vi "Create GUI Element.vi"(8 "error in (no error)":errorcluster, 10 "Highlight index":i32=-1, 11 "Sequence of SBlocks in":refnum<class "Sequence of SBlocks.lvclass">) -> (0 "error out":errorcluster, 2 "Sequence of SBlocks - GUI":T1, 3 "Sequence of SBlocks out":refnum<class "Sequence of SBlocks.lvclass">)   [LabVIEW 2020, in "TALOS.lvlib" / "Run Utilities.lvlib" / "Sequence of SBlocks.lvclass"]
uses:
  Sequence of SBlocks.lvclass
  Sequence of SBlcoks - GUI.ctl
  Schedule Block/Schedule Block - simplified GUI.ctl
  Sequence of SBlocks.lvclass/Sequence of SBlocks.ctl
  Schedule Block/Schedule Block.lvclass
panel:
  # "Estimated time of execution"
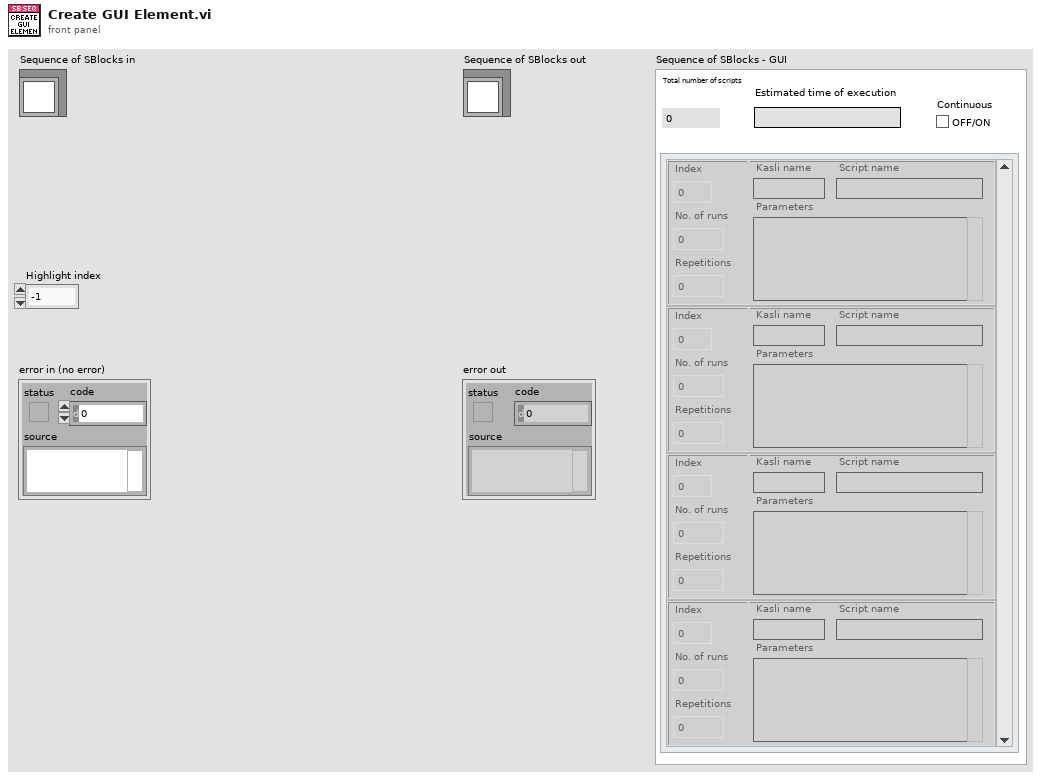
[diagram p1: front panel]
types:
  T1 = typedef "TALOS.lvlib/Run Utilities.lvlib/Sequence of SBlocks.lvclass/Sequence of SBlcoks - GUI.ctl" = cluster{"Total number of scripts":i32, "Time":string, "Sequence of SBlocks":T2[], "Continuous":bool}
  T2 = typedef "TALOS.lvlib/Run Utilities.lvlib/Schedule Block.lvclass/Schedule Block - simplified GUI.ctl" = cluster{"Bcg Color":u32, "Index":i32, "No. of runs":i32, "Script name":string, "Kasli name":string, "Parameters":string, "Repetitions":i32}
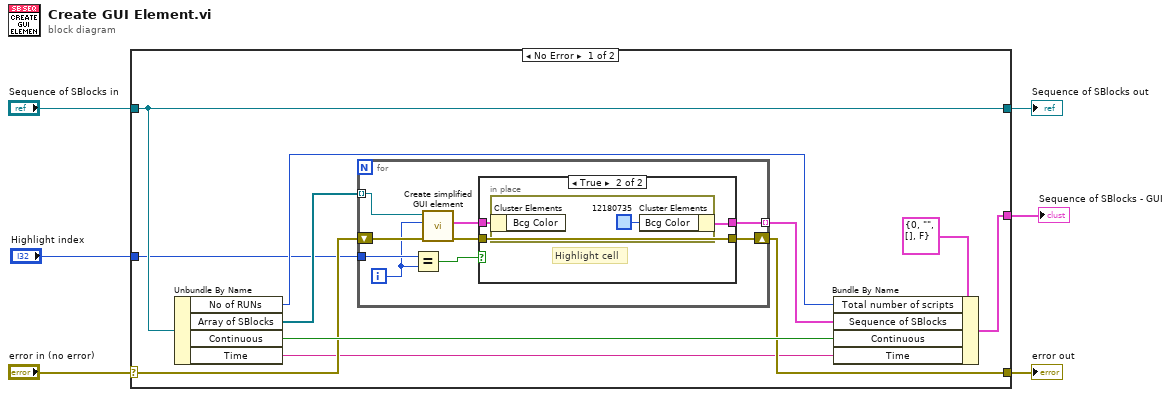
[diagram p0: block diagram]
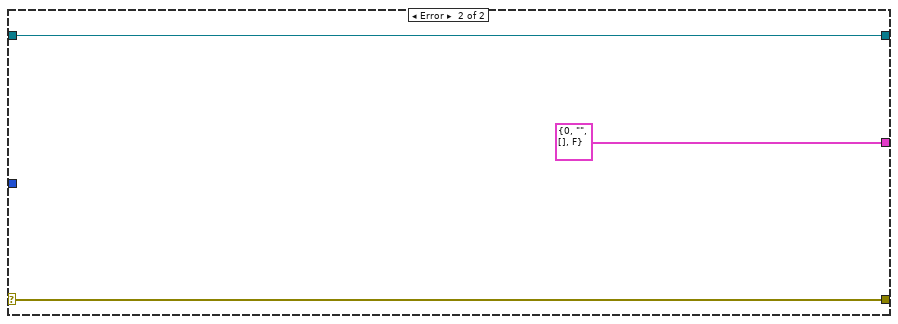
[diagram p3: hidden frame]
diagram:
  n1 = case shown="No Error" "error in (no error)" {
    selector: "error in (no error)" -> [w11 w35]
    tunnel: [w10 w35] -> w5
    tunnel: [w17 w34] -> w3
    tunnel: "Sequence of SBlocks in" -> [w17 w34]
    tunnel: [w12 T1 {"Total number of scripts"=0, "Time"="", "Sequence of SBlocks"=[], "Continuous"=FALSE} ("Sequence of SBlocks - GUI")] -> w2
    tunnel: "Highlight index" -> [w7 _]
    frame No Error {
      n2 = Unbundle By Name(w17) -> ("No of RUNs"=w9:i32, "Array of SBlocks"=w14:refnum<class "Schedule Block.lvclass">[], "Continuous"=w15:bool, "Time"=w8:string)
      n3 = for {
        tunnel: w14 -> [w25] mode=indexing
        tunnel: [w22] -> w13 mode=indexing
        shift-right: [w20] -> w10
        shift-left: w11 -> [w26]
        tunnel: w7 -> [w19]
        i -> [w18]
        n4 = Equal?(x=w19, y=w18) -> (x = y?=w24:bool)
        n5 = call-dynamic "Create simplified GUI element.vi"("error in (no error)"=w26, "Index"=w18, "Schedule Block in"=w25) -> ("error out"=w21:errorcluster, "Simple GUI Element"=w23:T2)  [unwired: 6 in, 1 out]
        n6 = case shown="True" w24 {
          tunnel: w23 -> [w28 w31]
          tunnel: [w28 w29] -> w22
          tunnel: w21 -> [w27 w30]
          tunnel: [w27 w30] -> w20
          frame False {
          }
          frame True {
            # "Highlight cell"
            n7 = in-place {
              n8 = in-place-cluster #1(w31) -> ()  [unwired: 1 out]
              n9 = in-place-cluster #1("Bcg Color"=u32 12180735) -> (w29:T2)
            }
          }
        }
      }
      n10 = Bundle By Name(cluster=T1 {"Total number of scripts"=0, "Time"="", "Sequence of SBlocks"=[], "Continuous"=FALSE} ("Sequence of SBlocks - GUI"), "Total number of scripts"=w9, "Sequence of SBlocks"=w13, "Continuous"=w15, "Time"=w8) -> (w12:T1)
    }
    frame Error {
    }
  }
  "error out" <- w5
  "Sequence of SBlocks out" <- w3
  "Sequence of SBlocks - GUI" <- w2
